vi "CheckWIPRecipe.vi"() -> ()   [LabVIEW 2012]
uses:
  <vilib>/addons/database/Auxilliary.llb/DB Tools Cursor Type.ctl
  <vilib>/addons/database/Connection.llb/DB Tools Open Connec (Path).vi
  <vilib>/addons/database/Connection.llb/Conn Execute.vi
  <vilib>/addons/database/Recordset.llb/Rec Fetch Recordset Data (R).vi
  <vilib>/addons/database/Recordset.llb/Rec Destroy - Connection.vi
  <vilib>/addons/database/_DB Variant To Data/Database Variant To Data.xnode
  <vilib>/addons/database/NI_Database_API.lvlib
panel:
  out "recordset data":variant[][](array[variant])
  out "error out":errorcluster
  out "spreadsheet string":string
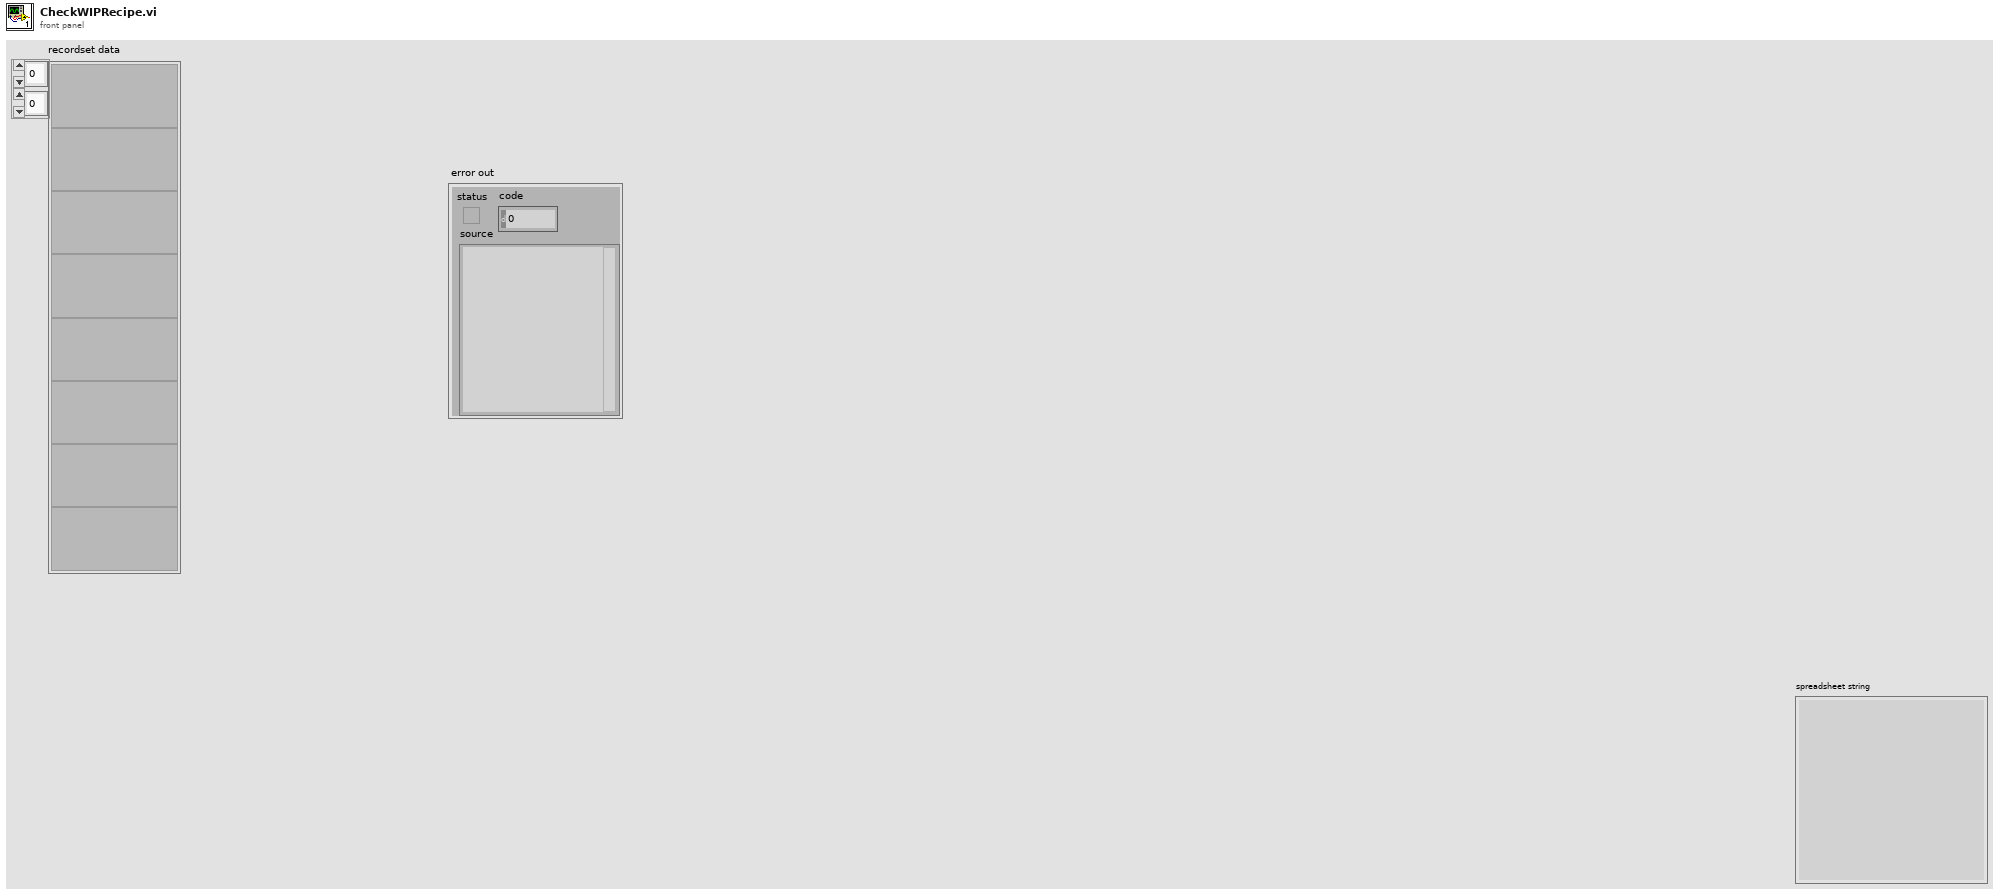
[diagram p1: front panel]
types:
  T1 = typedef "NI_Database_API.lvlib/DB Tools Cursor Type.ctl" = enum16{"forward-only", "keyset", "dynamic", "static"}
  T2 = typedef "NI_Database_API.lvlib/Conn ObjectReference.ctl" = refnum<k1>
  T3 = typedef "NI_Database_API.lvlib/Rec ObjectReference.ctl" = refnum<k1>
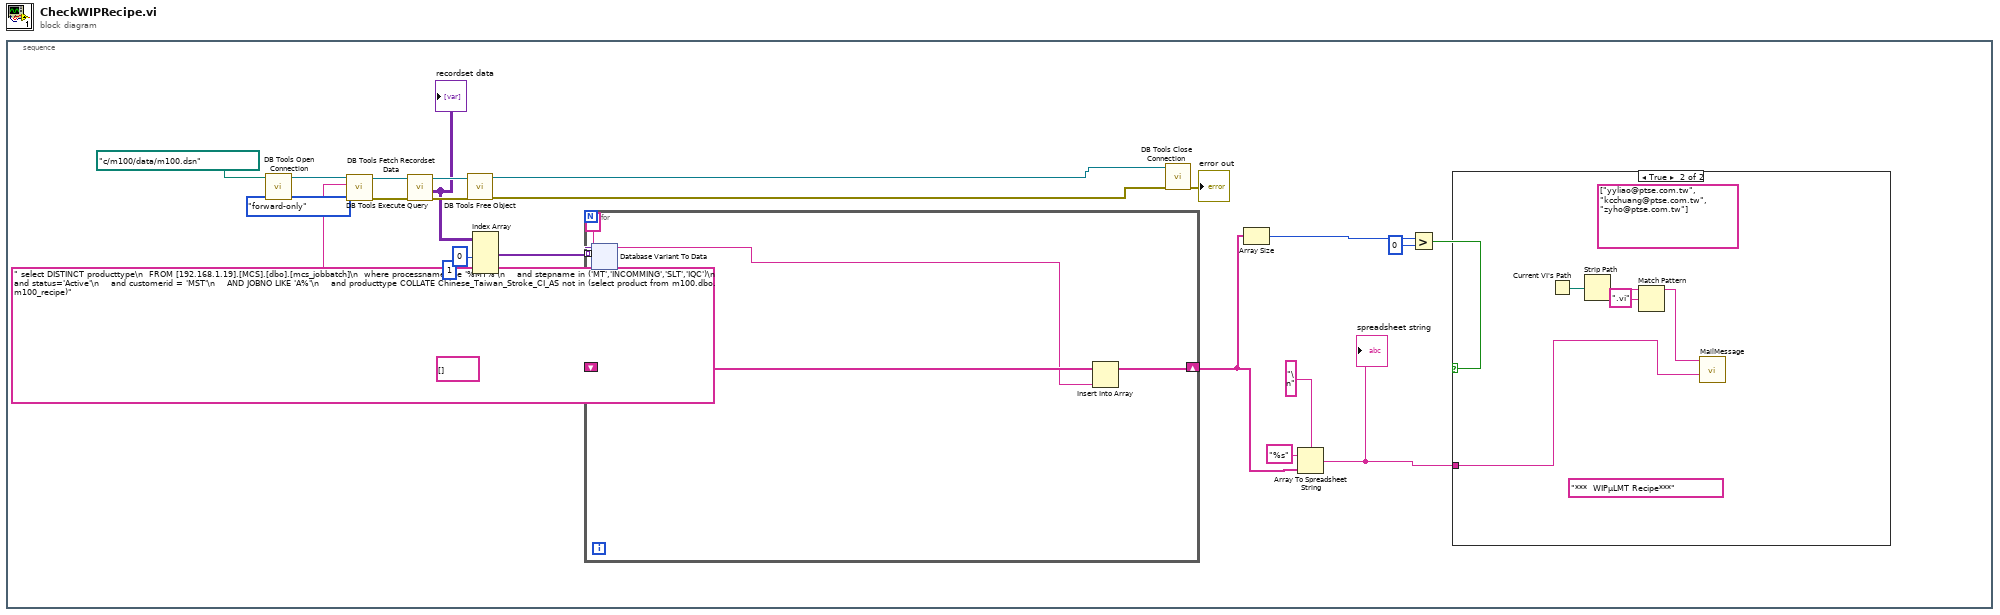
[diagram p0: block diagram]
diagram:
  n1 = stacked-sequence {
    frame #0 {
      n2 = call-poly <vilib>:"DB Tools Open Connection.vi"("connection information"=path "c:/m100/data/m100.dsn") -> ("error out"=w21:errorcluster, "connection reference"=w24:T2)  [unwired: 7 in]
      n3 = call-poly <vilib>:"DB Tools Execute Query.vi"("error in (no error)"=w21, "cursor type"=DB_Tools_Cursor_Type."forward-only", "SQL query"=" select DISTINCT producttype\n  FROM [192.168.1.19].[MCS].[dbo].[mcs_jobbatch]\n  where processname like '%MT%'\n    and stepname in ('MT','INCOMMING','SLT','IQC')\n    and status='Active'\n    and customerid = 'MST'\n    AND JOBNO LIKE 'A%'\n    and producttype COLLATE Chinese_Taiwan_Stroke_CI_AS not in (select product from m100.dbo.m100_recipe)", "connection reference"=w24) -> ("error out"=w20:errorcluster, "recordset reference"=w23:T3)  [unwired: 4 in]
      n4 = call-poly <vilib>:"DB Tools Fetch Recordset Data.vi"("error in (no error)"=w20, "recordset reference"=w23) -> ("error out"=w19:errorcluster, "recordset data"=w16:variant[][], "recordset reference out"=w22:T3)  [unwired: 3 in]
      "recordset data" <- w16
      n5 = call-poly <vilib>:"DB Tools Free Object.vi"("error in (no error)"=w19, "recordset reference"=w22) -> ("error out"=w1:errorcluster, "connection reference"=w2:T2)  [unwired: 8 in]
      n6 = Index Array(array=w16, index (col) #1=0 ("disabled index (col)"), index (col) #2=1 ("index (col)")) -> (element #1=w12:variant[])  [unwired: 2 in, 1 out]
      n7 = for {
        tunnel: w12 -> [w33] mode=indexing
        shift-right: [w32] -> w5
        shift-left: string[] [] ("array") -> [w31]
        n8 = xnode "Database Variant To Data"("database variant"=w33, "type"="") -> ("data"=w30:string)  [unwired: 1 in, 1 out]
        n9 = Insert Into Array(array=w31, new element=w30) -> (w32:string[])  [unwired: 1 in]
      }
      n10 = call <vilib>:"DB Tools Close Connection.vi"("error in (no error)"=w1, "connection reference"=w2) -> ("error out"=→"error out":errorcluster)  [unwired: 5 in]
      n11 = Array Size(array=w5) -> (size(s)=w4:i32)
      n12 = Array To Spreadsheet String(delimiter (Tab)="\n", array=w5, 3:"%s" ("format string")) -> (spreadsheet string=w7:string)
      "spreadsheet string" <- w7
      n13 = Greater?(x=w4, y=0) -> (0:w3:bool)
      n14 = case shown="True" w3 {
        tunnel: w7 -> [_ w25]
        frame False {
        }
        frame True {
          (unwired) "***  WIPµLMT Recipe***" ("subject ([No Subject])")
          (unwired) string[] ["yyliao@ptse.com.tw", "kcchuang@ptse.com.tw", "zyho@ptse.com.tw"] ("recipients")
          n15 = Current VI's Path() -> (path=w29:path)
          n16 = Strip Path(path=w29) -> (name=w28:string)  [unwired: 1 out]
          n17 = Match Pattern(string=w28, regular expression=".vi") -> (before substring=w26:string)  [unwired: 1 in, 3 out]
          n18 = call "MailMessage.vi"("message"=w25, "program"=w26) -> ()  [unwired: 10 in]
        }
      }
    }
  }
